vi "formatSweepResults.vi"(8 "error in (no error)":errorcluster, 10 "SweepResults":T1) -> (0 "error out":errorcluster, 1 "Wavenames":string[](array[string]), 2 "Data":cluster{"y":dbl[]}[](array[cluster]))   [LabVIEW 2016]
uses:
  LockinDAQ/Typedefs/SweepResults--Cluster.ctl
  LockinDAQ/LockinDAQ.lvclass
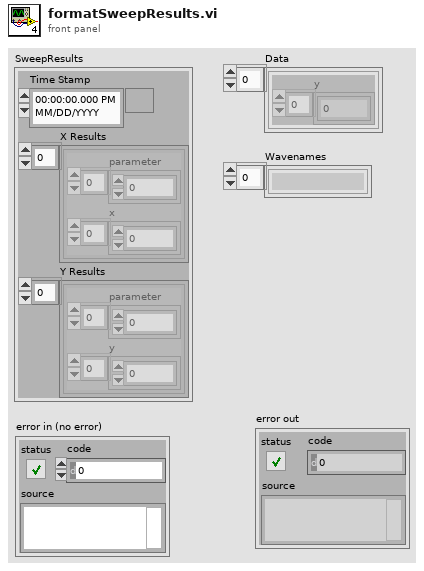
[diagram p1: front panel]
types:
  T1 = typedef "LockinDAQ.lvclass/SweepResults--Cluster.ctl" = cluster{"Time Stamp":timestamp, "X Results":cluster{"parameter":dbl[], "x":dbl[]}[], "Y Results":cluster{"parameter":dbl[], "y":dbl[]}[]}
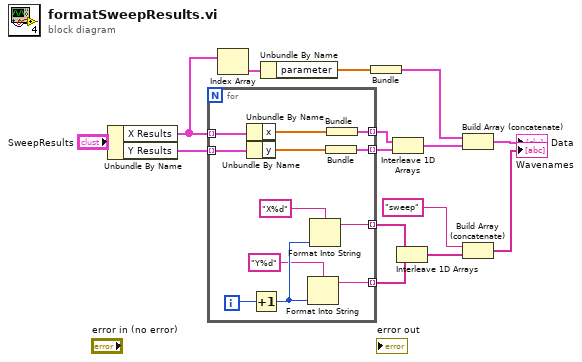
[diagram p0: block diagram]
diagram:
  n1 = Unbundle By Name("SweepResults") -> ("X Results"=w3:cluster{"parameter":dbl[], "x":dbl[]}[], "Y Results"=w4:cluster{"parameter":dbl[], "y":dbl[]}[])
  n2 = for {
    tunnel: w3 -> [w23] mode=indexing
    tunnel: [w27] -> w6 mode=indexing
    tunnel: [w25] -> w8 mode=indexing
    tunnel: w4 -> [w22] mode=indexing
    tunnel: [w19] -> w5 mode=indexing
    tunnel: [w16] -> w9 mode=indexing
    i -> [w26]
    n3 = Unbundle By Name(w23) -> ("x"=w21:dbl[])
    n4 = Unbundle By Name(w22) -> ("y"=w20:dbl[])
    n5 = Increment(x=w26) -> (x+1=w18:i32)
    n6 = Format Into String(format string="Y%d", w18) -> (resulting string=w16:string)  [unwired: 2 in, 1 out]
    n7 = Format Into String(format string="X%d", w18) -> (resulting string=w25:string)  [unwired: 2 in, 1 out]
    n8 = Bundle("y"=w20) -> (w19:cluster{"y":dbl[]})  [unwired: 1 in]
    n9 = Bundle("x"=w21) -> (w27:cluster{"x":dbl[]})  [unwired: 1 in]
  }
  n10 = Index Array(array=w3) -> (element=w1:cluster{"parameter":dbl[], "x":dbl[]})  [unwired: 1 in]
  n11 = Unbundle By Name(w1) -> ("parameter"=w2:dbl[])
  n12 = Bundle("parameter"=w2) -> (w14:cluster{"parameter":dbl[]})  [unwired: 1 in]
  n13 = Interleave 1D Arrays(w6, w5) -> (w7:cluster{"y":dbl[]}[])
  n14 = Interleave 1D Arrays(w8, w9) -> (w10:string[])
  n15 = Build Array (concatenate)(w14, w7) -> (→"Data":cluster{"y":dbl[]}[])
  n16 = Build Array (concatenate)("sweep" ("format string"), w10) -> (→"Wavenames":string[])
